vi "_Test_GetIDviaString.vi"() -> ()   [LabVIEW 2023]
uses:
  <vilib>/xnet/xnet.llb/XNET String To IO Name (Signal).vi
  <resource>/objmgr/xnet.rc
panel:
  out "Array":string[](array[string])
  out "Frame":refnum<k21>
  out "Name (Short)":string
  in  "string":string
  out "Identifier":u32
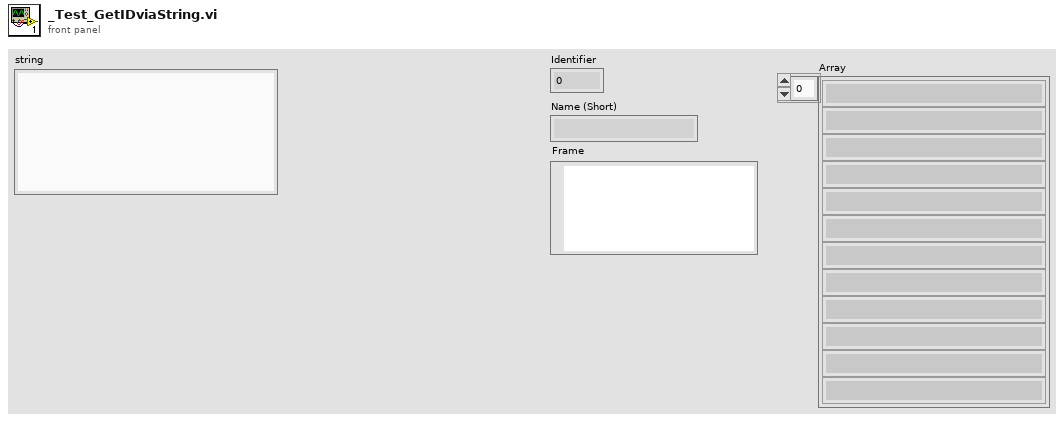
[diagram p1: front panel]
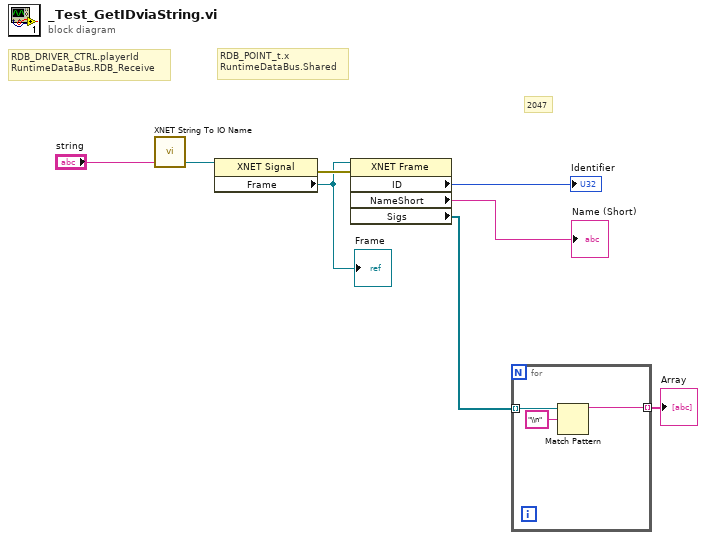
[diagram p0: block diagram]
diagram:
  # "RDB_POINT_t.x\nRuntimeDataBus.Shared"
  # "2047"
  # "RDB_DRIVER_CTRL.playerId\nRuntimeDataBus.RDB_Receive"
  n1 = call-poly <vilib>:"XNET String To IO Name.vi"("string"="string") -> ("XNET Signal"=w2:refnum<k21>)  [unwired: 4 out]
  n2 = property class="XNET Signal"(reference=w2) -> (error out=w8:errorcluster, "Frame"=w3:refnum<k21>)  [unwired: 1 in, 1 out]
  "Frame" <- w3
  n3 = property class="XNET Frame"(reference=w3, error in=w8) -> ("ID"=→"Identifier":u32, "NameShort"=→"Name (Short)":string, "Sigs"=w1:refnum<k21>[])  [unwired: 2 out]
  n4 = for {
    tunnel: w1 -> [w11] mode=indexing
    tunnel: [w9] -> w4 mode=indexing
    n5 = Match Pattern(string=w11, regular expression="\\n") -> (before substring=w9:string)  [unwired: 1 in, 3 out]
  }
  "Array" <- w4
